vi "sub_main_vlp16.vi"(8 "error in":errorcluster) -> (0 "error out":errorcluster)   [LabVIEW 2019]
uses:
  Ctrl/vlp-16 cmd.ctl
  Ctrl/error_modules.ctl
panel:
  out "vlp16 udp loop":i32
  out "main loop":i32
  out "err":bool
  out "receive data":string
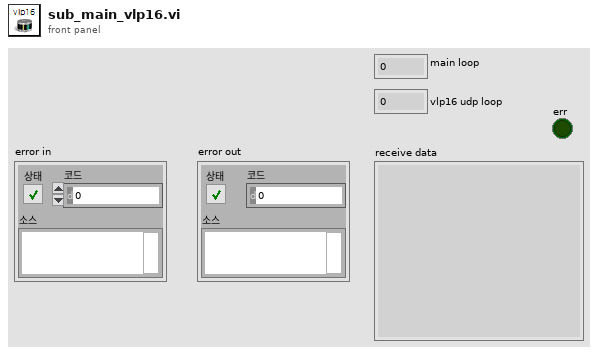
[diagram p1: front panel]
types:
  T1 = cluster{"id":i32, "arimuth(degree)":dbl, "vertical(degree)":dbl, "distance(meter)":dbl, "reflectivity":u8, "times(s)":ext, "x":dbl, "y":dbl, "z":dbl}[]
  T2 = typedef "error_modules.ctl" = enum16{"init", "read", "TIM571 error in", "VLP16 error in", "PwrPak7 error in"}
  T3 = typedef "vlp-16 cmd.ctl" = enum16{"write all data", "write xyz data", "read"}
  T4 = typedef "error_cluster.ctl" = cluster{"AGV":u16, "AGV Estop":u16, "Obstacle":u16, "Heading":u16, "Waypt":u16, "GNSS":u16, "VLP16":u16, "Cam":T5, "RPLidar":u16, "Joystick":u16, "IMU":T5}
  T5 = typedef "error_single-ring.ctl" = u8
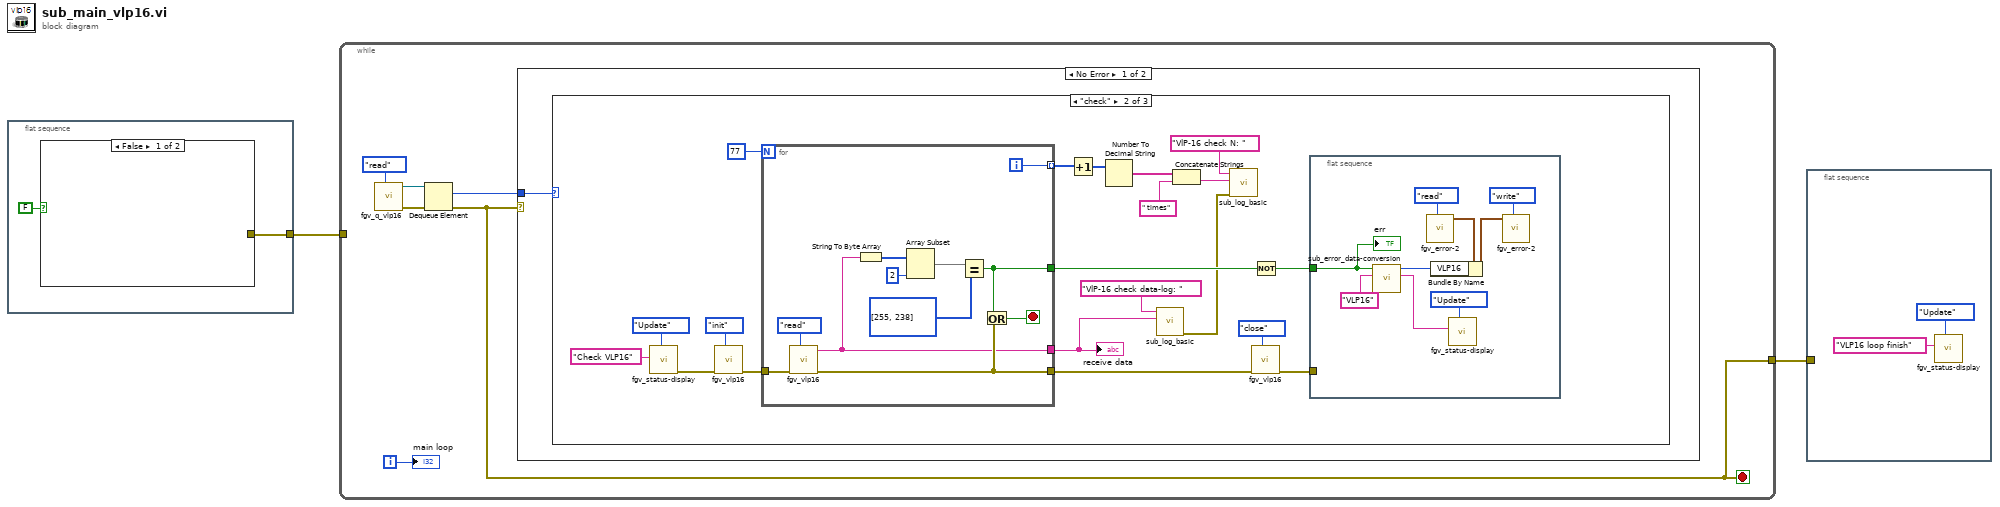
[diagram p0: block diagram]
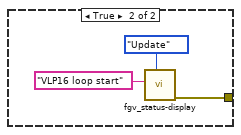
[diagram p2: hidden frame]
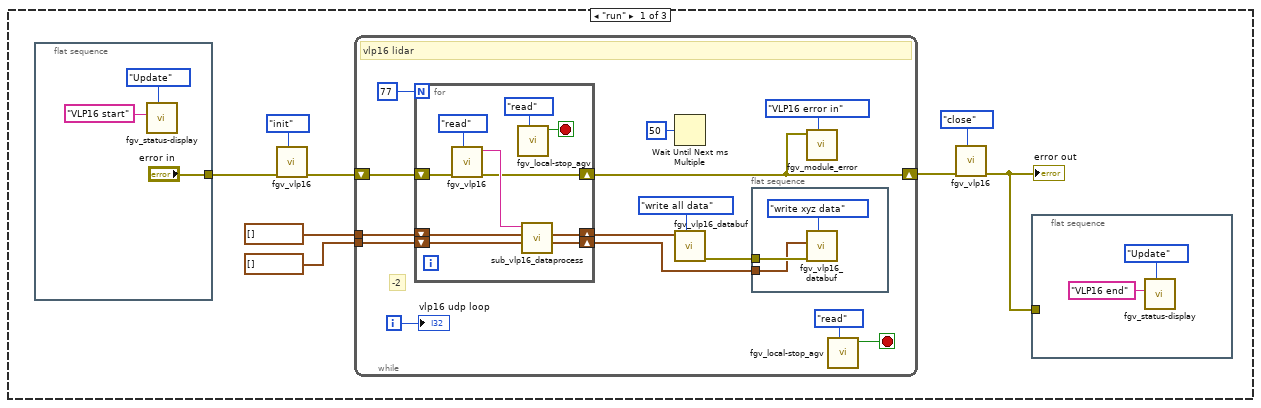
[diagram p3: hidden frame]
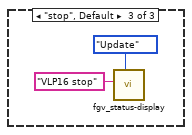
[diagram p4: hidden frame]
diagram:
  n1 = flat-sequence {
    tunnel: [w4] -> w1
    frame #0 {
      n2 = case shown="False" FALSE {
        tunnel: [_ w5] -> w4
        frame False {
        }
        frame True {
          n3 = call "fgv_status-display.vi"("Mode"=enum16{"Initial", "Update", "Clear"}."Update", "title"="VLP16 loop start" ("String in 1")) -> ("error out"=w5:errorcluster)  [unwired: 9 in]
        }
      }
    }
  }
  n4 = while {
    tunnel: [w9] -> w2
    tunnel: w1 -> [_]
    i -> [w8]
    stop <- w9 stop-if-true
    n5 = call "fgv_q_vlp16.vi"("cmd"=enum16{"create", "write", "read", "close"}."read") -> ("error out"=w11:errorcluster, "queue out"=w12:refnum<queue>)  [unwired: 9 in]
    n6 = Dequeue Element(queue=w12, error in (no error)=w11) -> (element=w10:enum16{"run", "check", "stop"}, error out=w9:errorcluster)  [unwired: 1 in, 2 out]
    n7 = case shown="No Error" w9 {
      tunnel: w10 -> [w14 _]
      frame No Error {
        n8 = case shown="\"check\"" w14 {
          frame "run" {
            n9 = flat-sequence {
              tunnel: ["error in"] -> w17
              frame #0 {
                n10 = call "fgv_status-display.vi"("Mode"=enum16{"Initial", "Update", "Clear"}."Update", "title"="VLP16 start" ("String in 1")) -> ()  [unwired: 9 in, 1 out]
              }
            }
            n11 = call "fgv_vlp16.vi"("cmd"=enum16{"init", "read", "write", "close"}."init", "error in"=w17) -> ("error out"=w20:errorcluster)  [unwired: 8 in, 1 out]
            n12 = while {
              shift-right: [w31] -> w16
              shift-left: w20 -> [w41]
              tunnel: T1 [] -> [w40]
              tunnel: cluster{"x":dbl, "y":dbl, "z":dbl}[] [] -> [w37]
              i -> [w29]
              stop <- w33 stop-if-true
              # "-2"
              # "vlp16 lidar"
              n13 = for {
                N: 77 -> [_]
                shift-right: [w51] -> w31
                shift-left: w41 -> [w49]
                shift-right: [w48] -> w32
                shift-left: w40 -> [w54]
                shift-right: [w47] -> w28
                shift-left: w37 -> [w52]
                stop <- w45 stop-if-true
                n14 = call "fgv_vlp16.vi"("cmd"=enum16{"init", "read", "write", "close"}."read", "error in"=w49) -> ("error out"=w51:errorcluster, "receive data"=w53:string)  [unwired: 8 in]
                n15 = call "fgv_local-stop_agv.vi"("cmd"=enum16{"ini", "read", "stop"}."read") -> ("stop status"=w45:bool)  [unwired: 10 in]
                n16 = call "sub_vlp16_dataprocess.vi"("data buf2"=w52, "data buf1"=w54, "receive data"=w53) -> ("xyz_data"=w47:cluster{"x":dbl, "y":dbl, "z":dbl}[], "all_data"=w48:T1)  [unwired: 7 in]
              }
              n17 = Wait Until Next ms Multiple(millisecond multiple=u32 50) -> ()  [unwired: 1 out]
              n18 = call "fgv_vlp16_databuf.vi"("cmd"=vlp-16_cmd."write all data", "raw data in"=w32) -> ("error out"=w35:errorcluster)  [unwired: 7 in, 2 out]
              n19 = flat-sequence {
                tunnel: w35 -> [w44]
                tunnel: w28 -> [w42]
                frame #0 {
                  n20 = call "fgv_vlp16_databuf.vi"("cmd"=vlp-16_cmd."write xyz data", "error in"=w44, "xyz_data"=w42) -> ()  [unwired: 6 in, 3 out]
                }
              }
              n21 = call "fgv_module_error.vi"("cmd"=error_modules."VLP16 error in", "vlp16 error in"=w31) -> ()  [unwired: 7 in, 3 out]
              n22 = call "fgv_local-stop_agv.vi"("cmd"=enum16{"ini", "read", "stop"}."read") -> ("stop status"=w33:bool)  [unwired: 10 in]
              "vlp16 udp loop" <- w29
            }
            n23 = call "fgv_vlp16.vi"("cmd"=enum16{"init", "read", "write", "close"}."close", "error in"=w16) -> ("error out"=w15:errorcluster)  [unwired: 8 in, 1 out]
            "error out" <- w15
            n24 = flat-sequence {
              tunnel: w15 -> [_]
              frame #0 {
                n25 = call "fgv_status-display.vi"("Mode"=enum16{"Initial", "Update", "Clear"}."Update", "title"="VLP16 end" ("String in 1")) -> ()  [unwired: 9 in, 1 out]
              }
            }
          }
          frame "check" {
            n26 = call "fgv_status-display.vi"("Mode"=enum16{"Initial", "Update", "Clear"}."Update", "title"="Check VLP16" ("String in 1")) -> ("error out"=w68:errorcluster)  [unwired: 9 in]
            n27 = call "fgv_vlp16.vi"("cmd"=enum16{"init", "read", "write", "close"}."init", "error in"=w68) -> ("error out"=w70:errorcluster)  [unwired: 8 in, 1 out]
            n28 = for {
              N: 77 -> [_]
              tunnel: w70 -> [w93]
              tunnel: [w87] -> w56
              tunnel: [w85] -> w60
              tunnel: [w88] -> w66
              tunnel: [w84] -> w61 mode=indexing
              i -> [w84]
              stop <- w86 stop-if-true
              n29 = call "fgv_vlp16.vi"("cmd"=enum16{"init", "read", "write", "close"}."read", "error in"=w93) -> ("error out"=w87:errorcluster, "receive data"=w85:string)  [unwired: 8 in]
              n30 = String To Byte Array(string=w85) -> (unsigned byte array=w92:u8[])
              n31 = Array Subset(array=w92, length=2) -> (w90:u8[])  [unwired: 1 in]
              n32 = Equal?(x=w90, y=u8[] [255, 238]) -> (x = y?=w88:bool)
              n33 = Or(x=w88, y=w87) -> (x .or. y?=w86:bool)
            }
            "receive data" <- w60
            n34 = Increment(x=w61) -> (x+1=w64:i32[])
            n35 = Number To Decimal String(number=w64) -> (decimal integer string=w63:string[])  [unwired: 1 in]
            n36 = call "sub_log_basic.vi"("desc"=w60, "Title"="VlP-16 check data-log: ") -> ("error out"=w55:errorcluster)  [unwired: 9 in]
            n37 = Concatenate Strings(w63, " times" ("문자열")) -> (w57:string)
            n38 = call "sub_log_basic.vi"("error in"=w55, "desc"=w57, "Title"="VlP-16 check N: ") -> ()  [unwired: 8 in, 1 out]
            n39 = call "fgv_vlp16.vi"("cmd"=enum16{"init", "read", "write", "close"}."close", "error in"=w56) -> ("error out"=w67:errorcluster)  [unwired: 8 in, 1 out]
            n40 = Not(x=w66) -> (.not. x?=w65:bool)
            n41 = flat-sequence {
              tunnel: w65 -> [w75]
              tunnel: w67 -> [_]
              frame #0 {
                n42 = call "sub_error_data-conversion.vi"("name"="VLP16", "error status"=w75) -> ("check result string"=w76:string, "error conversion out"=w83:u16)  [unwired: 8 in]
                n43 = call "fgv_error-2.vi"("cmd"=enum16{"init", "read", "write"}."read") -> ("Error cluster out"=w82:T4)  [unwired: 9 in, 1 out]
                n44 = Bundle By Name(cluster=w82, "VLP16"=w83) -> (w81:T4)
                n45 = call "fgv_status-display.vi"("Mode"=enum16{"Initial", "Update", "Clear"}."Update", "title"=w76) -> ()  [unwired: 9 in, 1 out]
                n46 = call "fgv_error-2.vi"("cmd"=enum16{"init", "read", "write"}."write", "Error cluster"=w81) -> ()  [unwired: 8 in, 2 out]
                "err" <- w75
              }
            }
          }
          frame "stop", Default {
            n47 = call "fgv_status-display.vi"("Mode"=enum16{"Initial", "Update", "Clear"}."Update", "title"="VLP16 stop" ("String in 1")) -> ()  [unwired: 9 in, 1 out]
          }
        }
      }
      frame Error {
      }
    }
    "main loop" <- w8
  }
  n48 = flat-sequence {
    tunnel: w2 -> [_]
    frame #0 {
      n49 = call "fgv_status-display.vi"("Mode"=enum16{"Initial", "Update", "Clear"}."Update", "title"="VLP16 loop finish" ("String in 1")) -> ()  [unwired: 9 in, 1 out]
    }
  }
